vi "Toggle IO Enable.vi"(8 "error in":errorcluster, 10 "IO_EN":bool, 11 "SL_SC in":refnum<class "SL_SC.lvclass">) -> (0 "error out":errorcluster, 3 "SL_SC out":refnum<class "SL_SC.lvclass">)   [LabVIEW 2019, in "SL_SC.lvlib" / "SL_SC.lvclass"]
doc: "This VI Is provided in support of the SLSC Chassis operation where the outputs can be enabled/disabled as a protection for flight hardware."
uses:
  Library/SL_SC.lvclass
  Library/SL_SC.lvclass/SL_SC.ctl
  <vilib>/SLSC/Set Device Property (I32).vi
  <vilib>/SLSC/Commit Properties for Devices.vi
  builds/Instruments/DIG_IO.lvlibp/Library/DIG_IO.lvclass
  <vilib>/SLSC/SLSC.lvlib
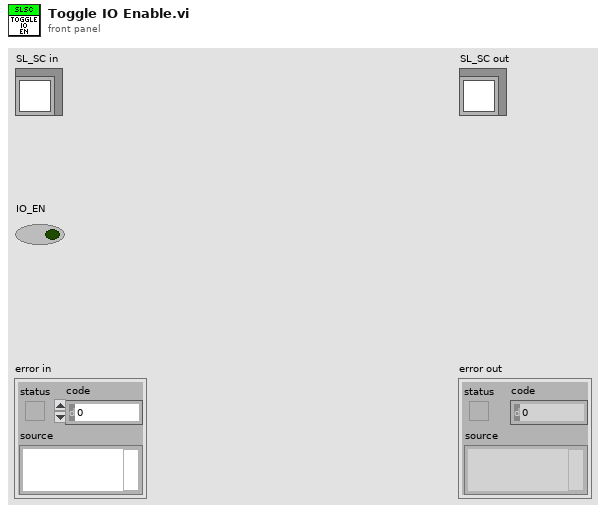
[diagram p1: front panel]
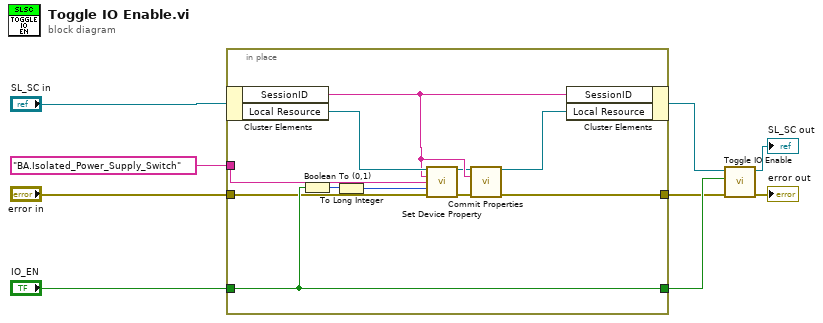
[diagram p0: block diagram]
diagram:
  n1 = in-place {
    in-place-border: "error in" -> [w13]
    in-place-border: "BA.Isolated_Power_Supply_Switch" -> [w17]
    in-place-border: "IO_EN" -> [w16]
    in-place-border: [w16] -> w2
    in-place-border: [w12] -> w1
    n2 = in-place-cluster #1("SL_SC in") -> ("SessionID"=w19:string, "Local Resource"=w20:refnum<k21>)
    n3 = Boolean To (0,1)(Boolean=w16) -> (0, 1=w15:i16)
    n4 = To Long Integer(number=w15) -> (32bit integer=w14:i32)
    n5 = call-poly <vilib>:"Set Device Property.vi"("session in"=w20, "devices"=w19, "property"=w17, "property value"=w14, "error in (no error)"=w13) -> ("session out"=w10:refnum<k21>, "error out"=w11:errorcluster)  [unwired: 9 in]
    n6 = call-poly <vilib>:"Commit Properties.vi"("session in"=w10, "devices"=w19, "error in (no error)"=w11) -> ("session out"=w18:refnum<k21>, "error out"=w12:errorcluster)  [unwired: 11 in]
    n7 = in-place-cluster #1("SessionID"=w19, "Local Resource"=w18) -> (w5:refnum<class "SL_SC.lvclass">)
  }
  n8 = call-parent "Toggle IO Enable.vi"("error in"=w1, "IO_EN"=w2, "DIG_IO in"=w5) -> ("error out"=→"error out":errorcluster, "DIG_IO out"=→"SL_SC out":refnum<class "SL_SC.lvclass">)  [unwired: 7 in]
